vi "Change Padding.vi"(8 "error in (no error)":errorcluster, 10 "Padding":T1 caption="HLP_just/pad", 11 "Numeric Data Type in":refnum<class "Numeric Data Type.lvclass">) -> (0 "error out":errorcluster, 3 "Numeric Data Type out":refnum<class "Numeric Data Type.lvclass">)   [LabVIEW 2018, in "Numeric Data Type.lvclass"]
uses:
  Numeric Data Type.lvclass
  Padding.ctl
  Numeric Data Type.lvclass/Numeric Data Type.ctl
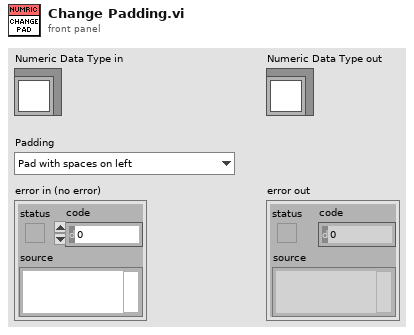
[diagram p1: front panel]
types:
  T1 = typedef "Numeric Data Type.lvclass/Padding.ctl" = enum16{"Pad with spaces on left", "Pad with spaces on right", "Pad with zeros on left"}
  T2 = typedef "Numeric Data Type.lvclass/Numeric Info.ctl" = cluster{"Minimum Field Width":i32, "Digits of Precision":i32, "Numeric Format":T3, "Precision Type":T4, "Hide trailing zeros":bool, "exponent":bool, "just/pad":T1, "Modifiers":string}
  T3 = typedef "Numeric Data Type.lvclass/Numeric Format Enum.ctl" = enum16{"Floating Point Notation", "Scientific Notation", "Engineering Notation", "SI Notation", "<not used>", "Decimal", "Hexadecimal", "Octal", "Binary", "<not used 2>", "Absolute Time", "Relative Time"}
  T4 = typedef "Numeric Data Type.lvclass/Precision Type.ctl" = enum16{"Digits of precision", "Significant digits"}
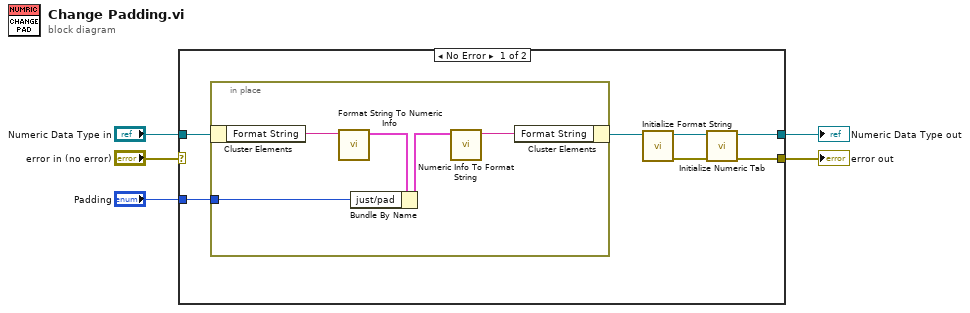
[diagram p0: block diagram]
diagram:
  n1 = case shown="No Error" "error in (no error)" {
    selector: "error in (no error)" -> [_ w19]
    tunnel: [w7 w19] -> w4
    tunnel: [w9 w18] -> w2
    tunnel: "Numeric Data Type in" -> [w12 w18]
    tunnel: "Padding" -> [w6 _]
    frame No Error {
      n2 = in-place {
        in-place-border: w6 -> [w13]
        n3 = in-place-cluster #1(w12) -> ("Format String"=w17:string)
        n4 = call "Format String To Numeric Info.vi"("Format String"=w17) -> ("Numeric Format & Precision Info"=w16:T2)  [unwired: 10 in]
        n5 = Bundle By Name(cluster=w16, "just/pad"=w13) -> (w15:T2)
        n6 = call "Numeric Info To Format String.vi"("Numeric Format & Precision Info"=w15) -> ("Format String"=w14:string)  [unwired: 10 in]
        n7 = in-place-cluster #1("Format String"=w14) -> (w11:refnum<class "Numeric Data Type.lvclass">)
      }
      n8 = call "Initialize Format String.vi"("Numeric Data Type in"=w11) -> ("error out"=w8:errorcluster, "Numeric Data Type (dup)"=w10:refnum<class "Numeric Data Type.lvclass">)  [unwired: 9 in]
      n9 = call "Initialize Numeric Tab.vi"("error in (no error)"=w8, "Numeric Data Type in"=w10) -> ("error out"=w7:errorcluster, "Numeric Data Type (dub)"=w9:refnum<class "Numeric Data Type.lvclass">)  [unwired: 8 in]
    }
    frame Error {
    }
  }
  "error out" <- w4
  "Numeric Data Type out" <- w2
